vi "FGV Interference.vi"(0 "TestKonfig":T5={"Komponente:"=0, "Modus"=0, "CG Aufschaltzeit:"=120.0, "Interferent 1:"=0, "Interferent 2:"=0, "Interferent 3:"=0, "Gasflaschen Nr.:"="", "Gasflaschen Nr.: 2"="", "Gasflaschen Nr.: 3"="", "Inter 1 aktiv"=FALSE, "Inter 2 aktiv"=FALSE, "Inter 3 aktiv"=FALSE, "Accuracy"="", "Accuracy 2"="", "Accuracy 3"="", "Konzentration 1:"=120.0, "Konzentration 2:"=120.0, "Konzentration 3:"=120.0} {"Konzentration 3:" min=0.0; "Konzentration 2:" min=0.0; "Konzentration 1:" min=0.0; "Modus" items=["Messen", "CG zu Entnahmestelle"]; "CG Aufschaltzeit:" min=60.0}, 1 "TestSetting":T1={"Bearbeiter:"="", "Pfad:"=path "D:/IAG_Data/Log", "Textname:"="", "Analysator"=""}, 5 "Ergebnis":sgl[](array[numeric]), 7 "Êinheiten":string[](array[string]), 9 "Tabelle":T3[][](array[typedef]), 11 "error in (no error)":errorcluster caption="Fehler (Eingang, kein Fehler)", 12 "Aktion FGV Interference":T7) -> (3 "TestSetting":T1={"Bearbeiter:"="", "Pfad:"=path "D:/IAG_Data/Log", "Textname:"="", "Analysator"=""}, 4 "TestKonfig 2":T5={"Komponente:"=0, "Modus"=0, "CG Aufschaltzeit:"=120.0, "Interferent 1:"=0, "Interferent 2:"=0, "Interferent 3:"=0, "Gasflaschen Nr.:"="", "Gasflaschen Nr.: 2"="", "Gasflaschen Nr.: 3"="", "Inter 1 aktiv"=FALSE, "Inter 2 aktiv"=FALSE, "Inter 3 aktiv"=FALSE, "Accuracy"="", "Accuracy 2"="", "Accuracy 3"="", "Konzentration 1:"=120.0, "Konzentration 2:"=120.0, "Konzentration 3:"=120.0} {"Konzentration 3:" min=0.0; "Konzentration 2:" min=0.0; "Konzentration 1:" min=0.0; "Modus" items=["Messen", "CG zu Entnahmestelle"]; "CG Aufschaltzeit:" min=60.0}, 6 "Ergebnis":T4, 8 "Êinheiten":string[](array[string]), 10 "Tabelle":T3[][](array[typedef]), 15 "error out":errorcluster caption="Fehler (Ausgang)")   [LabVIEW 2020, in "EPA 1065.lvlib" / "Interference verificaton 1065-375.lvlib"]
uses:
  Interference verificaton 1065-375.lvlib
  Aktion FGV Interference.ctl
  TestKonfig.ctl
  Modus.ctl
  Ergebnis.ctl
  Visualisierungs Elemente/String - Ausgabefeld.ctl
  TestSetting.ctl
  Seiten/System Einstellungen V2/Analysatoren.ctl
  Linearisierung V2/AktivButton.ctl
  Allgemein/allgemeine Sub-VIs.lvlib
  Linearisierung V2/Linearisierung v2.lvlib
  Seiten/System Einstellungen V2/System Einstellungen V2.lvlib
panel:
  in  "Ergebnis":T4 caption="Cluster"
  # "sec."
  # "sec."
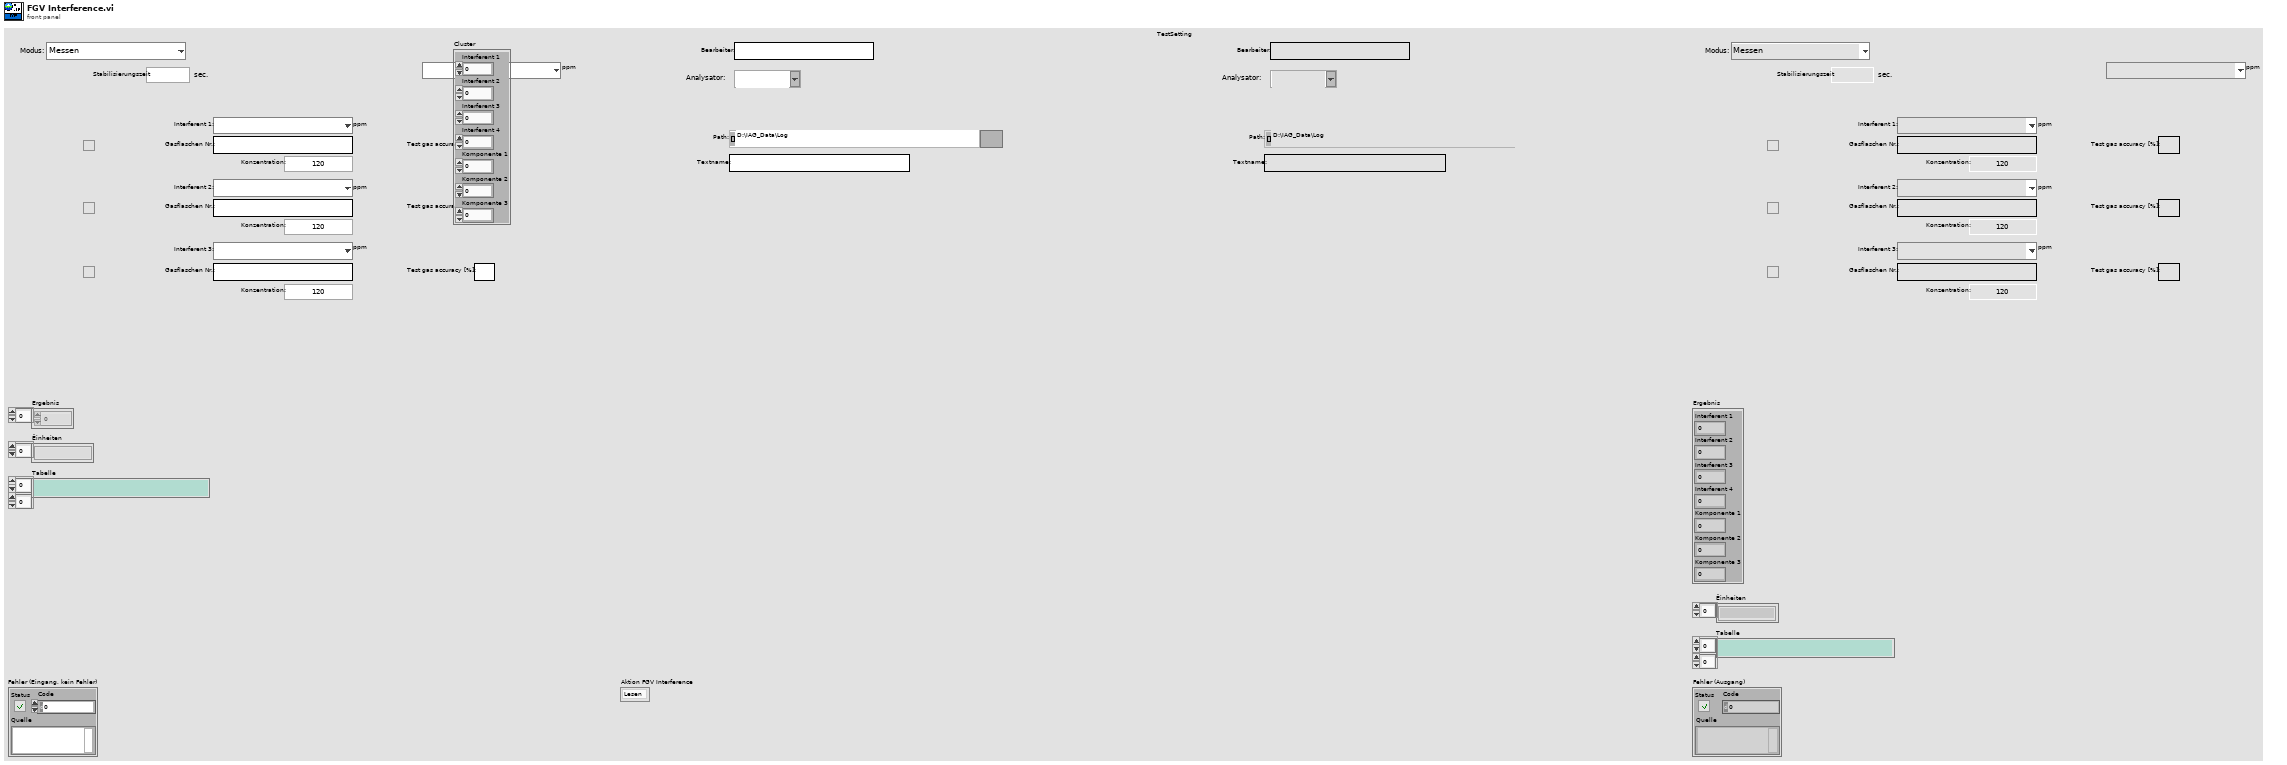
[diagram p1: front panel]
types:
  T1 = typedef "EPA 1065.lvlib/Interference verificaton 1065-375.lvlib/TestSetting.ctl" = cluster{"Bearbeiter:":string, "Pfad:":path, "Textname:":string, "Analysator":T2}
  T2 = typedef "System Einstellungen V2.lvlib/Analysatoren.ctl" = string
  T3 = typedef "String - Ausgabefeld.ctl" = string
  T4 = typedef "EPA 1065.lvlib/Interference verificaton 1065-375.lvlib/Ergebnis.ctl" = cluster{"Interferent 1":sgl, "Interferent 2":sgl, "Interferent 3":sgl, "Interferent 4":sgl, "Komponente 1":sgl, "Komponente 2":sgl, "Komponente 3":sgl}
  T5 = typedef "EPA 1065.lvlib/Interference verificaton 1065-375.lvlib/TestKonfig.ctl" = cluster{"Komponente:":u16, "Modus":T6, "CG Aufschaltzeit:":dbl, "Interferent 1:":u16, "Interferent 2:":u16, "Interferent 3:":u16, "Gasflaschen Nr.:":string, "Gasflaschen Nr.: 2":string, "Gasflaschen Nr.: 3":string, "Inter 1 aktiv":bool, "Inter 2 aktiv":bool, "Inter 3 aktiv":bool, "Accuracy":string, "Accuracy 2":string, "Accuracy 3":string, "Konzentration 1:":dbl, "Konzentration 2:":dbl, "Konzentration 3:":dbl}
  T6 = typedef "EPA 1065.lvlib/Interference verificaton 1065-375.lvlib/Modus.ctl" = u16
  T7 = typedef "EPA 1065.lvlib/Interference verificaton 1065-375.lvlib/Aktion FGV Interference.ctl" = enum16{"Lesen", "TestKonfig", "TestSetting", "Einheiten", "Ergebnis", "Laden", "Tabelle", "Speichern", "löschen"}
  T8 = enum16{"open", "replace", "create", "open or create", "replace or create", "replace or create with confirmation"}
  T9 = typedef "Linearisierung v2.lvlib/AktivButton.ctl" = bool
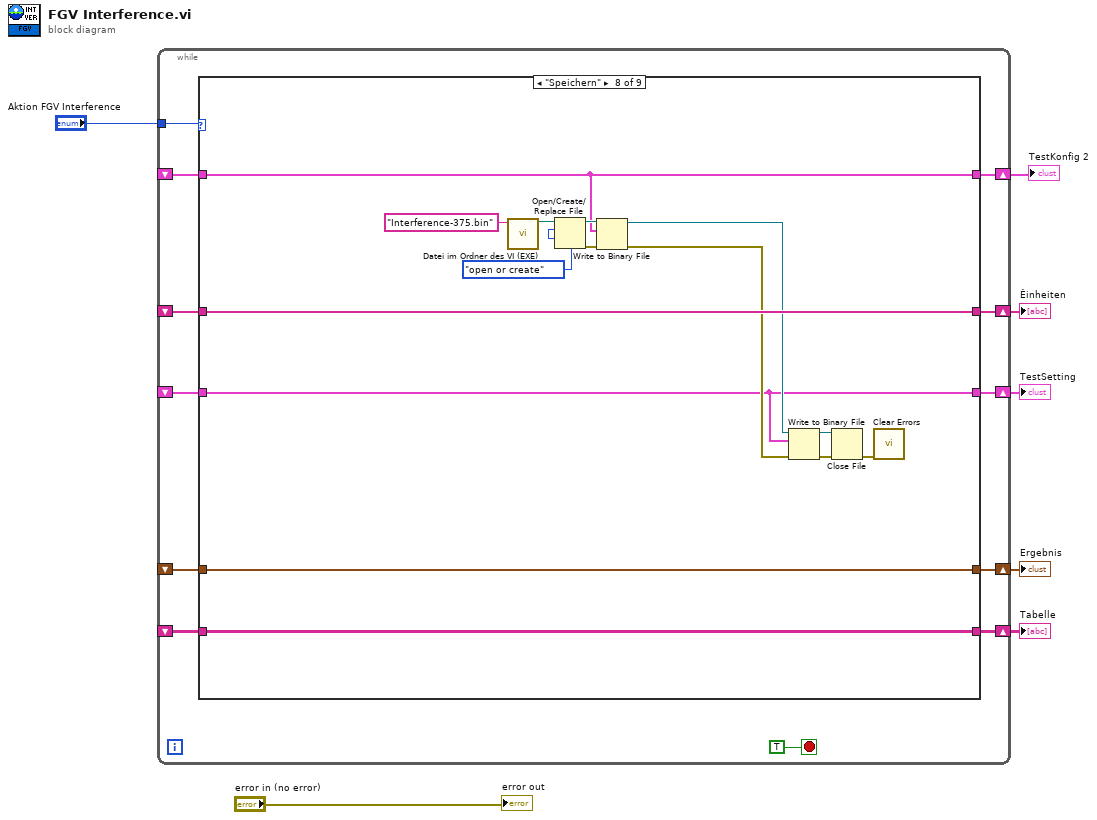
[diagram p0: block diagram]
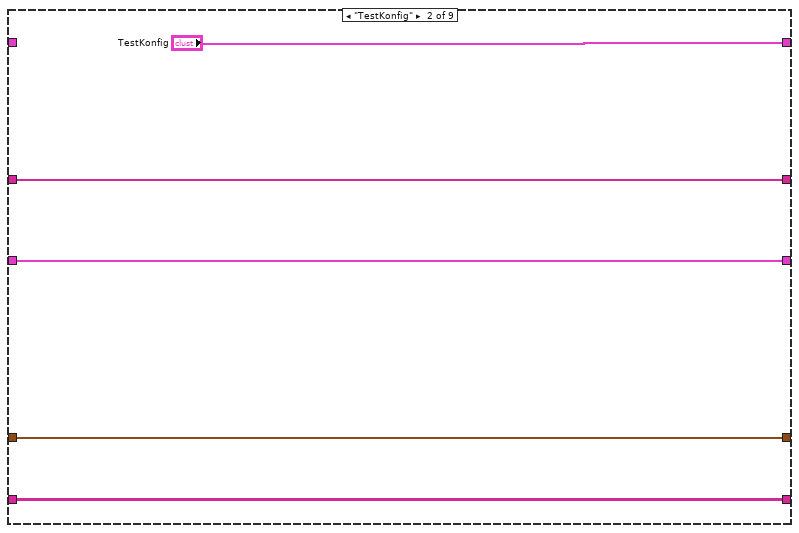
[diagram p3: hidden frame]
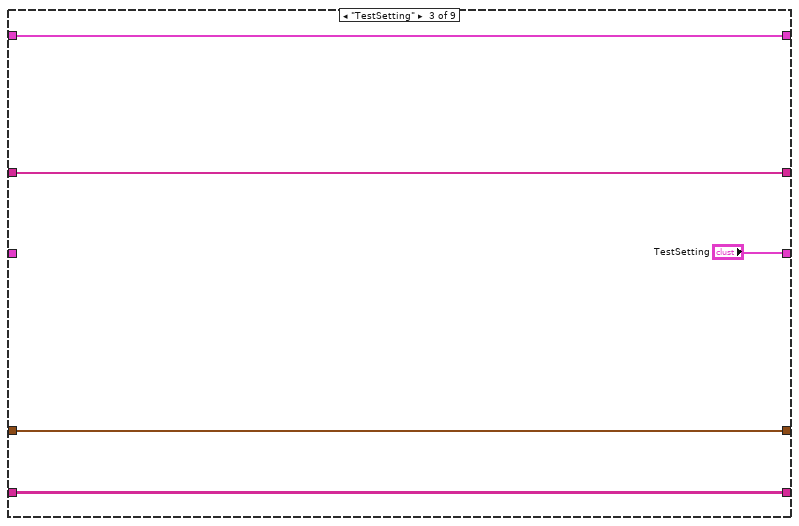
[diagram p4: hidden frame]
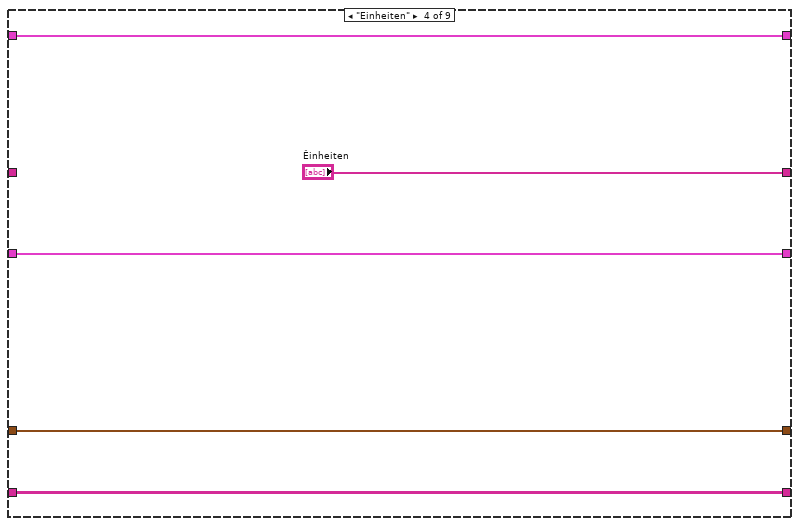
[diagram p5: hidden frame]
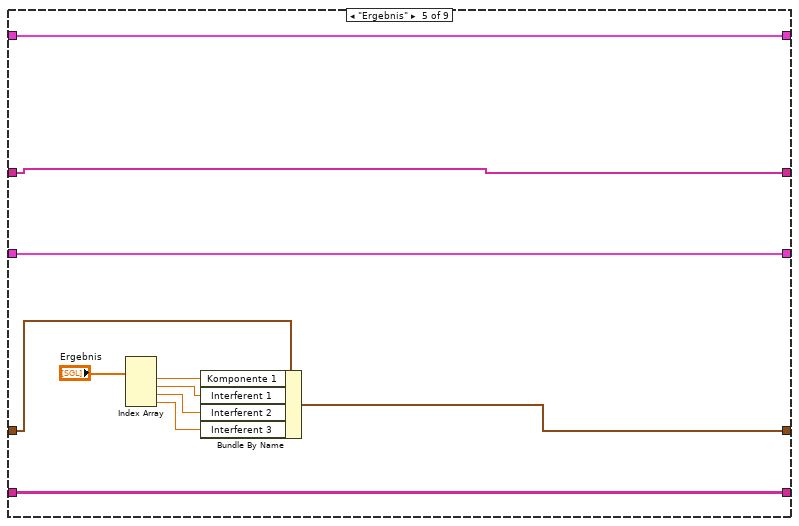
[diagram p6: hidden frame]
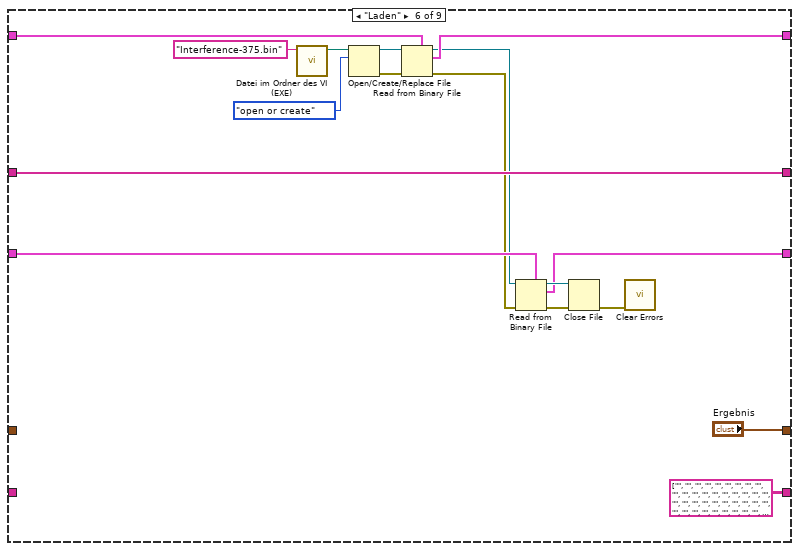
[diagram p7: hidden frame]
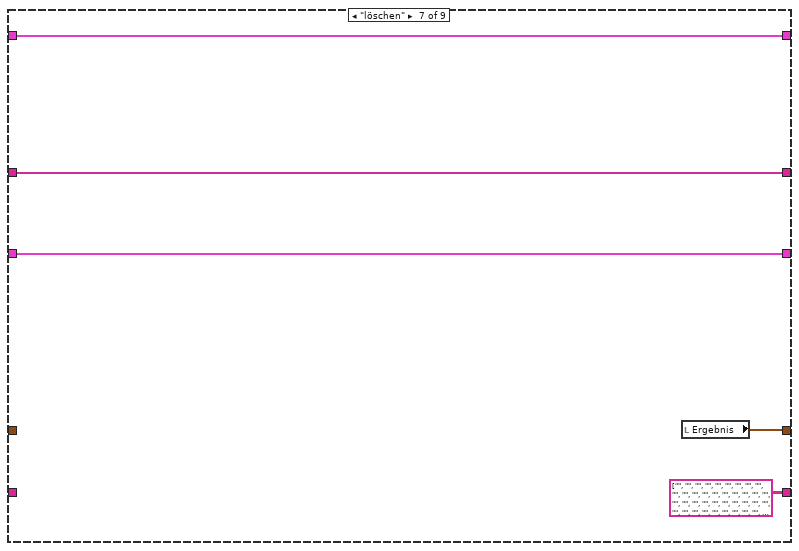
[diagram p8: hidden frame]
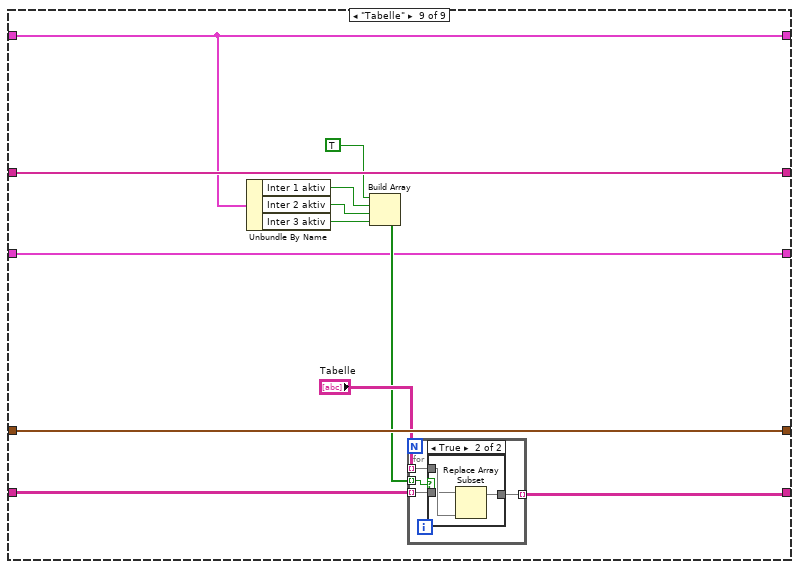
[diagram p9: hidden frame]
diagram:
  n1 = while {
    tunnel: "Aktion FGV Interference" -> [w18]
    shift-right: [w19] -> w5
    shift-left: _ -> [w17]
    shift-right: [w15] -> w4
    shift-left: _ -> [w14]
    shift-right: [w13] -> w3
    shift-left: _ -> [w12]
    shift-right: [w11] -> w2
    shift-left: _ -> [w10]
    shift-right: [w9] -> w1
    shift-left: _ -> [w8]
    stop <- TRUE stop-if-true
    n2 = case shown="\"Speichern\"" w18 {
      tunnel: [w24 "TestKonfig" w31 w39 w50 w58 w70 w79 w97] -> w19
      tunnel: w17 -> [w24 _ w31 w39 w50 w59 w70 w79 w97]
      tunnel: [w23 w28 w34 w38 w41 "Ergebnis" w69 w87 w99] -> w15
      tunnel: w14 -> [w23 w28 w34 w38 w48 _ _ w87 w99]
      tunnel: [w22 w27 w33 "Êinheiten" w47 w66 w72 w86 w98] -> w13
      tunnel: w12 -> [w22 w27 w33 _ w47 w66 w72 w86 w98]
      tunnel: [w21 w26 w32 w36 w46 T3[][] [["", "", "", "", "", "", "", "", "", "", ""], ["", "", "", "", "", "", "", "", "", "", ""], ["", "", "", "", "", "", "", "", "", "", ""], ["", "", "", "", "", "", "", "", "", "", ""], ["", "", "", "", "", "", "", "", "", "", ""], ["", "", "", "", "", "", "", "", "", "", ""], ["", "", "", "", "", "", "", "", "", "", ""], ["", "", "", "", "", "", "", "", "", "", ""], ["", "", "", "", "", "", "", "", "", "", ""], ["", "", "", "", "", "", "", "", "", "", ""], ["", "", "", "", "", "", "", "", "", "", ""]] ("Tabelle") T3[][] [["", "", "", "", "", "", "", "", "", "", ""], ["", "", "", "", "", "", "", "", "", "", ""], ["", "", "", "", "", "", "", "", "", "", ""], ["", "", "", "", "", "", "", "", "", "", ""], ["", "", "", "", "", "", "", "", "", "", ""], ["", "", "", "", "", "", "", "", "", "", ""], ["", "", "", "", "", "", "", "", "", "", ""], ["", "", "", "", "", "", "", "", "", "", ""], ["", "", "", "", "", "", "", "", "", "", ""], ["", "", "", "", "", "", "", "", "", "", ""], ["", "", "", "", "", "", "", "", "", "", ""]] ("Tabelle") w85 w94] -> w11
      tunnel: w10 -> [w21 w26 w32 w36 w46 _ _ w85 w95]
      tunnel: [w20 w25 "TestSetting" w35 w40 w53 w68 w73 w89] -> w9
      tunnel: w8 -> [w20 w25 _ w35 w40 w54 w68 w73 w89]
      frame "Lesen", Default {
      }
      frame "TestKonfig" {
      }
      frame "TestSetting" {
      }
      frame "Einheiten" {
      }
      frame "Ergebnis" {
        n3 = Index Array(array="Ergebnis") -> (element #1=w45:sgl, element #2=w44:sgl, element #3=w43:sgl, element #4=w42:sgl)  [unwired: 4 in]
        n4 = Bundle By Name(cluster=w48, "Komponente 1"=w45, "Interferent 1"=w44, "Interferent 2"=w43, "Interferent 3"=w42) -> (w41:T4)
      }
      frame "Laden" {
        n5 = call "Datei im Ordner des VI (EXE).vi"("Dateiname"="Interference-375.bin") -> ("Dateipfad im Ordner des Haupt-VIs"=w63:path)  [unwired: 8 in, 2 out]
        n6 = Open/Create/Replace File(file path (use dialog)=w63, operation (0:open)=T8."open or create" ("Operation (0:open)")) -> (refnum out=w61:refnum<file>, error out=w62:errorcluster)  [unwired: 4 in, 1 out]
        n7 = Read from Binary File(5:w59, 8:w62, 11:w61) -> (0:w51:errorcluster, 2:w58:T5, 3:w52:refnum<file>)  [unwired: 3 in, 1 out]
        n8 = Read from Binary File(5:w54, 8:w51, 11:w52) -> (0:w55:errorcluster, 2:w53:T1, 3:w57:refnum<file>)  [unwired: 3 in, 1 out]
        n9 = Close File(refnum=w57, error in=w55) -> (error out=w56:errorcluster)  [unwired: 1 out]
        n10 = call <vilib>:"Clear Errors.vi"("error in (no error)"=w56) -> ()  [unwired: 5 in, 2 out]
      }
      frame "löschen" {
        n11 = local read "Ergebnis"() -> (w69:T4)
      }
      frame "Speichern" {
        n12 = call "Datei im Ordner des VI (EXE).vi"("Dateiname"="Interference-375.bin") -> ("Dateipfad im Ordner des Haupt-VIs"=w83:path)  [unwired: 8 in, 2 out]
        n13 = Open/Create/Replace File(file path (use dialog)=w83, operation (0:open)=T8."open or create" ("Operation (0:open)")) -> (refnum out=w84:refnum<file>, error out=w82:errorcluster)  [unwired: 4 in, 1 out]
        n14 = Write to Binary File(file (use dialog)=w84, data=w79, error in=w82) -> (refnum out=w75:refnum<file>, error out=w74:errorcluster)  [unwired: 3 in, 1 out]
        n15 = Write to Binary File(file (use dialog)=w75, data=w73, error in=w74) -> (refnum out=w77:refnum<file>, error out=w78:errorcluster)  [unwired: 3 in, 1 out]
        n16 = Close File(refnum=w77, error in=w78) -> (error out=w76:errorcluster)  [unwired: 1 out]
        n17 = call <vilib>:"Clear Errors.vi"("error in (no error)"=w76) -> ()  [unwired: 5 in, 2 out]
      }
      frame "Tabelle" {
        n18 = Unbundle By Name(w97) -> ("Inter 1 aktiv"=w93:bool, "Inter 2 aktiv"=w92:bool, "Inter 3 aktiv"=w88:bool)
        n19 = Build Array(T9 TRUE ("Element"), w93, w92, w88) -> (w91:T9[])
        n20 = for {
          tunnel: "Tabelle" -> [w103] mode=indexing
          tunnel: w95 -> [w102] mode=indexing
          tunnel: [w101] -> w94 mode=indexing
          tunnel: w91 -> [w100] mode=indexing
          n21 = case shown="True" w100 {
            tunnel: w103 -> [_ w107]
            tunnel: w102 -> [w104 w106]
            tunnel: [w104 w105] -> w101
            frame False {
            }
            frame True {
              n22 = Replace Array Subset(array=w106, new element=w107) -> (w105:T3[])  [unwired: 1 in]
            }
          }
        }
      }
    }
  }
  "TestKonfig 2" <- w5
  "Ergebnis" <- w4
  "Êinheiten" <- w3
  "Tabelle" <- w2
  "TestSetting" <- w1
  "error out" <- "error in (no error)"
